vi "observacao_queued.vi"() -> ()   [LabVIEW 2012, in "Shared_160.lvlib"] (continued)
                    n1496 = Get Date/Time In Seconds() -> (seconds since 1Jan1904=w1913:timestamp)
                    n1497 = Add(x=w1913, y=10.0) -> (x+y=w1914:timestamp)
                    n1498 = property on="WeakSel" class="Bool (strict)"("Value"=w1910) -> ()  [unwired: 2 in, 2 out]
                    n1499 = property on="Weak" class="Bool (strict)"("Value"=w1910) -> ()  [unwired: 2 in, 2 out]
                    n1500 = local write "alarm Time"(w1914) -> ()
                    n1501 = property on="Mensage Alarme" class="Str"("Visible"=TRUE) -> ()  [unwired: 2 in, 2 out]
                    n1502 = local write "Flag Alarm"(TRUE ("Flag Alarm")) -> ()
                  }
                }
              }
              event "Medium": Value Change {
                w1917 = u16 6 items=["Alarme", "Atencao", "Erro", "Ocupado", "TBD", "LCB", "Trapeira", "Paravento", "DomoRap", "DomoCW", "DomoCCW", "TBD", "Em movimento", "TBD"] ("NomeStatus")
                n1503 = event-data() -> ("NewVal"=w1918:bool)  [unwired: 1 in, 5 out]
                n1504 = call "Bit Status CUP.vi"("NomeStatus"=w1917) -> ("StatBit"=w1916:bool)
                n1505 = case shown="False" w1916 {
                  tunnel: w1918 -> [w1925 _]
                  frame False {
                    w1920 = u16 4 items=["ZERO", "AH", "DEC", "TUBO", "CUP"] ("Controlador")
                    n1506 = case shown="True" w1925 {
                      tunnel: [0 2] -> w1922
                      tunnel: [w1927 TRUE] -> w1923
                      tunnel: [w1927 FALSE] -> w1921
                      tunnel: ["DESLIGAR" "LIGAR"] -> w1924
                      frame False {
                        w1927 = FALSE
                      }
                      frame True {
                        n1507 = local write "DOME"(FALSE) -> ()
                        n1508 = local write "StatShutter"("Busy to Close" ("Status")) -> ()
                      }
                    }
                    n1509 = property on="Weak" class="Bool (strict)"("Disabled"=w1922) -> ()  [unwired: 2 in, 2 out]
                    n1510 = property on="Strong" class="Bool (strict)"("Disabled"=w1922) -> ()  [unwired: 2 in, 2 out]
                    n1511 = property on="WeakSel" class="Bool (strict)"("Value"=w1921) -> ()  [unwired: 2 in, 2 out]
                    n1512 = property on="MediumSel" class="Bool (strict)"("Value"=w1923) -> ()  [unwired: 2 in, 2 out]
                    n1513 = property on="StrongSel" class="Bool (strict)"("Value"=w1921) -> ()  [unwired: 2 in, 2 out]
                    n1514 = property on="Coude" class="Bool (strict)"("DisabledEnum"=w1922) -> ()  [unwired: 2 in, 2 out]
                    n1515 = property on="CoudeSel" class="Bool (strict)"("Value"=w1921) -> ()  [unwired: 2 in, 2 out]
                    n1516 = call "Monta Comando.vi"("Comando"=w1924, "Dispositivo"="FLAT_LO", "Controlador"=w1920) -> ()  [unwired: 4 in, 3 out]
                  }
                  frame True {
                    w1935 = FALSE ("Medium")
                    n1517 = Get Date/Time In Seconds() -> (seconds since 1Jan1904=w1938:timestamp)
                    n1518 = Add(x=w1938, y=10.0) -> (x+y=w1939:timestamp)
                    n1519 = local write "alarm Time"(w1939) -> ()
                    n1520 = property on="Mensage Alarme" class="Str"("Visible"=TRUE) -> ()  [unwired: 2 in, 2 out]
                    n1521 = local write "Flag Alarm"(TRUE ("Flag Alarm")) -> ()
                    n1522 = property on="Medium" class="Bool (strict)"("Value"=w1935) -> ()  [unwired: 2 in, 2 out]
                    n1523 = property on="MediumSel" class="Bool (strict)"("Value"=w1935) -> ()  [unwired: 2 in, 2 out]
                  }
                }
              }
              event "Strong": Value Change {
                w1942 = u16 6 items=["Alarme", "Atencao", "Erro", "Ocupado", "TBD", "LCB", "Trapeira", "Paravento", "DomoRap", "DomoCW", "DomoCCW", "TBD", "Em movimento", "TBD"] ("NomeStatus")
                n1524 = event-data() -> ("NewVal"=w1943:bool)  [unwired: 1 in, 5 out]
                n1525 = call "Bit Status CUP.vi"("NomeStatus"=w1942) -> ("StatBit"=w1941:bool)
                n1526 = case shown="False" w1941 {
                  tunnel: w1943 -> [w1951 _]
                  frame False {
                    w1944 = u16 4 items=["ZERO", "AH", "DEC", "TUBO", "CUP"] ("Controlador")
                    n1527 = case shown="True" w1951 {
                      tunnel: [FALSE w1959] -> w1946
                      tunnel: [w1952 w1959] -> w1950
                      tunnel: [0 2] -> w1947
                      tunnel: ["DESLIGAR" "LIGAR"] -> w1949
                      tunnel: [w1952 TRUE] -> w1948
                      frame False {
                        w1952 = FALSE
                      }
                      frame True {
                        w1959 = FALSE
                        n1528 = local write "DOME"(FALSE) -> ()
                        n1529 = local write "StatShutter"("Busy to Close" ("Status")) -> ()
                      }
                    }
                    n1530 = property on="Medium" class="Bool (strict)"("Disabled"=w1947) -> ()  [unwired: 2 in, 2 out]
                    n1531 = property on="Weak" class="Bool (strict)"("Disabled"=w1947) -> ()  [unwired: 2 in, 2 out]
                    n1532 = property on="Coude" class="Bool (strict)"("DisabledEnum"=w1947) -> ()  [unwired: 2 in, 2 out]
                    n1533 = property on="WeakSel" class="Bool (strict)"("Value"=w1950) -> ()  [unwired: 2 in, 2 out]
                    n1534 = property on="MediumSel" class="Bool (strict)"("Value"=w1946) -> ()  [unwired: 2 in, 2 out]
                    n1535 = property on="StrongSel" class="Bool (strict)"("Value"=w1948) -> ()  [unwired: 2 in, 2 out]
                    n1536 = property on="CoudeSel" class="Bool (strict)"("Value"=w1946) -> ()  [unwired: 2 in, 2 out]
                    n1537 = call "Monta Comando.vi"("Comando"=w1949, "Dispositivo"="FLAT_HI", "Controlador"=w1944) -> ()  [unwired: 4 in, 3 out]
                  }
                  frame True {
                    w1962 = FALSE ("Strong")
                    n1538 = Get Date/Time In Seconds() -> (seconds since 1Jan1904=w1965:timestamp)
                    n1539 = Add(x=w1965, y=10.0) -> (x+y=w1966:timestamp)
                    n1540 = local write "alarm Time"(w1966) -> ()
                    n1541 = property on="Mensage Alarme" class="Str"("Visible"=TRUE) -> ()  [unwired: 2 in, 2 out]
                    n1542 = local write "Flag Alarm"(TRUE ("Flag Alarm")) -> ()
                    n1543 = property on="StrongSel" class="Bool (strict)"("Value"=w1962) -> ()  [unwired: 2 in, 2 out]
                    n1544 = property on="Strong" class="Bool (strict)"("Value"=w1962) -> ()  [unwired: 2 in, 2 out]
                  }
                }
              }
              event "Coude": Value Change {
                w1969 = u16 6 items=["Alarme", "Atencao", "Erro", "Ocupado", "TBD", "LCB", "Trapeira", "Paravento", "DomoRap", "DomoCW", "DomoCCW", "TBD", "Em movimento", "TBD"] ("NomeStatus")
                n1545 = event-data() -> ("NewVal"=w1970:bool)  [unwired: 1 in, 5 out]
                n1546 = call "Bit Status CUP.vi"("NomeStatus"=w1969) -> ("StatBit"=w1968:bool)
                n1547 = case shown="False" w1968 {
                  tunnel: w1970 -> [w1977 _]
                  frame False {
                    w1971 = u16 4 items=["ZERO", "AH", "DEC", "TUBO", "CUP"] ("Controlador")
                    n1548 = case shown="True" w1977 {
                      tunnel: [FALSE w1986] -> w1974
                      tunnel: [w1979 w1986] -> w1975
                      tunnel: [0 2] -> w1973
                      tunnel: ["DESLIGAR" "LIGAR"] -> w1978
                      tunnel: [w1979 TRUE] -> w1976
                      frame False {
                        w1979 = FALSE
                      }
                      frame True {
                        w1986 = FALSE
                        n1549 = local write "DOME"(FALSE) -> ()
                        n1550 = local write "StatShutter"("Busy to Close" ("Status")) -> ()
                      }
                    }
                    n1551 = property on="StrongSel" class="Bool (strict)"("Value"=w1975) -> ()  [unwired: 2 in, 2 out]
                    n1552 = property on="CoudeSel" class="Bool (strict)"("Value"=w1976) -> ()  [unwired: 2 in, 2 out]
                    n1553 = property on="MediumSel" class="Bool (strict)"("Value"=w1974) -> ()  [unwired: 2 in, 2 out]
                    n1554 = property on="Weak" class="Bool (strict)"("DisabledEnum"=w1973) -> ()  [unwired: 2 in, 2 out]
                    n1555 = property on="Medium" class="Bool (strict)"("DisabledEnum"=w1973) -> ()  [unwired: 2 in, 2 out]
                    n1556 = property on="Strong" class="Bool (strict)"("DisabledEnum"=w1973) -> ()  [unwired: 2 in, 2 out]
                    n1557 = property on="WeakSel" class="Bool (strict)"("Value"=w1974) -> ()  [unwired: 2 in, 2 out]
                    n1558 = call "Monta Comando.vi"("Comando"=w1978, "Dispositivo"="FLAT_COUDE", "Controlador"=w1971) -> ()  [unwired: 4 in, 3 out]
                  }
                  frame True {
                    w1989 = FALSE ("Coude")
                    n1559 = Get Date/Time In Seconds() -> (seconds since 1Jan1904=w1992:timestamp)
                    n1560 = Add(x=w1992, y=10.0) -> (x+y=w1993:timestamp)
                    n1561 = local write "alarm Time"(w1993) -> ()
                    n1562 = property on="Mensage Alarme" class="Str"("Visible"=TRUE) -> ()  [unwired: 2 in, 2 out]
                    n1563 = local write "Flag Alarm"(TRUE ("Flag Alarm")) -> ()
                    n1564 = property on="CoudeSel" class="Bool (strict)"("Value"=w1989) -> ()  [unwired: 2 in, 2 out]
                    n1565 = property on="Coude" class="Bool (strict)"("Value"=w1989) -> ()  [unwired: 2 in, 2 out]
                  }
                }
              }
            }
            n1566 = disable-structure shown="Disabled" {
              frame Disabled {
                w1889 = u16 4 items=["ZERO", "AH", "DEC", "TUBO", "CUP"] ("Controlador")
                n1567 = call "Monta Comando.vi"("Comando"="FECHAR", "Dispositivo"="TRAPEIRA" ("Comando"), "Controlador"=w1889) -> ()  [unwired: 4 in, 3 out]
              }
              frame Enabled {
              }
            }
          }
          frame "LIST" {
            n1568 = stacked-sequence {
              frame #0 {
                # "Muda nome do controle de RA para AH se MAFmax == 100"
                n1569 = case shown="True" "SET coord" {
                  frame False {
                  }
                  frame True {
                    n1570 = stacked-sequence {
                      frame #0 {
                        w2010 = "2000"
                        # "Valores aux para Detectar Edição"
                        n1571 = local read "Multicolumn Listbox"() -> (w2017:i32[])
                        n1572 = property on="Multicolumn Listbox" class="MCListbox (strict)"() -> ("Item Names"=w2015:string[][])  [unwired: 2 in, 2 out]
                        n1573 = Index Array(array=w2017, index=0) -> (element=w2014:i32)
                        n1574 = local write "FLAG SET COORD"(TRUE ("FLAG_MAG")) -> ()
                        n1575 = Index Array(array=w2015, index (row)=w2014) -> (element=w2013:string[])  [unwired: 1 in]
                        n1576 = Index Array(array=w2013, index #1=0 ("index")) -> (element #1=w2006:string, element #2=w2004:string, element #3=w2005:string, element #4=w2007:string, element #5=w2009:string, element #6=w2008:string)  [unwired: 5 in]
                        "RA AUX" <- w2004
                        "AUX EDITA Name" <- w2006
                        "AUX EDITA RA" <- w2004
                        "AUX EDITA DEC" <- w2005
                        "AUX EDITA PMRA" <- w2009
                        "AUX EDITA PMDEC" <- w2008
                        n1577 = local write "StrPointObjPMRA"(w2009) -> ()
                        n1578 = local write "StrPointObjPMDEC"(w2008) -> ()
                        n1579 = local write "StrPointObjName"(w2006) -> ()
                        n1580 = local write "StrPointObjRA"(w2004) -> ()
                        n1581 = local write "StrPointObjDEC"(w2005) -> ()
                        n1582 = local write "MAG"(w2007) -> ()
                        n1583 = local write "StrPointObjEpoch"(w2010) -> ()
                        "EPOCH AUX" <- w2010
                        "AUX EDITA EPOCH" <- w2010
                      }
                      frame #1 {
                        n1584 = case shown="True" "Case Constant\n(See Context Help) 7" {
                          frame False {
                          }
                          frame True {
                            # "Ao clicar SET COORD, fechar a aba LIST e abrir a aba POINTING"
                            n1585 = local write "Setup, Pointing & Guiding"(T2."POINTING" ("Setup, Pointing & Guiding")) -> ()
                          }
                        }
                      }
                    }
                  }
                }
                n1586 = case shown="True" "Clear ALL" {
                  frame False {
                  }
                  frame True {
                    n1587 = Two Button Dialog(message="Will you clear All Table?") -> (T button?=w2020:bool)  [unwired: 2 in]
                    n1588 = case shown="True" w2020 {
                      frame False {
                      }
                      frame True {
                        w2022 = string[][] [] ("Item Names")
                        # "Limpa a Tabela Inteira"
                        n1589 = property on="Multicolumn Listbox" class="MCListbox (strict)"("Item Names"=w2022) -> ()  [unwired: 2 in, 2 out]
                        n1590 = local write "subarray"(w2022) -> ()
                      }
                    }
                  }
                }
                n1591 = local read "MAG Max"() -> (w1996:dbl)
                n1592 = Equal?(x=100.0, y=w1996) -> (x = y?=w1995:bool)
                n1593 = case shown="False" w1995 {
                  frame False {
                    n1594 = flat-sequence {
                      frame #0 {
                        w2000 = FALSE
                        n1595 = property on="RA Max" class="DigNum (strict)"("Caption.Visible"=w2000) -> ()  [unwired: 2 in, 2 out]
                        n1596 = property on="RA Min" class="DigNum (strict)"("Caption.Visible"=w2000) -> ()  [unwired: 2 in, 2 out]
                      }
                      frame #1 {
                        w2001 = TRUE
                        n1597 = property on="RA Min" class="DigNum (strict)"("Label.Visible"=w2001) -> ()  [unwired: 2 in, 2 out]
                        n1598 = property on="RA Max" class="DigNum (strict)"("Label.Visible"=w2001) -> ()  [unwired: 2 in, 2 out]
                      }
                    }
                  }
                  frame True {
                    n1599 = flat-sequence {
                      frame #0 {
                        w2002 = FALSE
                        n1600 = property on="RA Max" class="DigNum (strict)"("Label.Visible"=w2002) -> ()  [unwired: 2 in, 2 out]
                        n1601 = property on="RA Min" class="DigNum (strict)"("Label.Visible"=w2002) -> ()  [unwired: 2 in, 2 out]
                      }
                      frame #1 {
                        w2003 = TRUE
                        n1602 = property on="RA Min" class="DigNum (strict)"("Caption.Visible"=w2003) -> ()  [unwired: 2 in, 2 out]
                        n1603 = property on="RA Max" class="DigNum (strict)"("Caption.Visible"=w2003) -> ()  [unwired: 2 in, 2 out]
                      }
                    }
                  }
                }
              }
              frame #1 {
                # "MUDANÇA:\nUPLOAD carrega\ncatálogo usuário"
                n1604 = case shown="True" "Upload" {
                  frame False {
                  }
                  frame True {
                    n1605 = File Dialog() -> (0:w2028:errorcluster, 1:w2030:bool, 3:w2029:path)  [unwired: 7 in, 1 out]
                    n1606 = Unbundle(w2028) -> ("status"=w2027:bool)  [unwired: 2 out]
                    n1607 = Not(x=w2027) -> (.not. x?=w2025:bool)
                    n1608 = And(x=w2030, y=w2025) -> (x .and. y?=w2026:bool)
                    n1609 = case shown="False" w2026 {
                      tunnel: w2029 -> [w2033 _]
                      frame False {
                        w2034 = 0 ("Slide")
                        # "Abre Arquivo Escolhido"
                        n1610 = Strip Path(path=w2033) -> (name=w2031:string)  [unwired: 1 out]
                        n1611 = Path To String(path=w2033) -> (string=w2038:string)
                        n1612 = local write "List File"(w2031) -> ()
                        n1613 = call "leexel.vi"("path"=w2038) -> ("array 5"=w2032:string[][])  [unwired: 4 in]
                        n1614 = local write "Slide"(w2034) -> ()
                        n1615 = local write "subarray"(w2032) -> ()
                        n1616 = Array Subset(array=w2032, index (row)=w2034, length (row)=10 ("length"), index (col)=w2034, length (col)=8 ("index")) -> (w2035:string[][])
                        n1617 = property on="Multicolumn Listbox" class="MCListbox (strict)"("Item Names"=w2035) -> ()  [unwired: 2 in, 2 out]
                      }
                      frame True {
                      }
                    }
                  }
                }
                n1618 = case shown="True" "Save AS" {
                  frame False {
                  }
                  frame True {
                    n1619 = File Dialog() -> (0:w2039:errorcluster, 1:w2041:bool, 3:w2040:path)  [unwired: 7 in, 1 out]
                    n1620 = Unbundle(w2039) -> ()  [unwired: 3 out]
                    n1621 = case shown="False" w2041 {
                      tunnel: w2040 -> [w2043 _]
                      frame False {
                        # "Salva Arquivo Escolhido"
                        n1622 = Path To String(path=w2043) -> (string=w2044:string)
                        n1623 = case shown="True" "Case Constant\n(See Context Help) 8" {
                          tunnel: w2044 -> [_ w2046]
                          frame False {
                          }
                          frame True {
                            n1624 = local read "subarray"() -> (w2045:string[][])
                            n1625 = call "salvaexel.vi"("appended array"=w2045, "file name p/ exell"=w2046) -> ()  [unwired: 1 in, 1 out]
                          }
                        }
                      }
                      frame True {
                      }
                    }
                  }
                }
              }
              frame #2 {
                # "Acerta Posição do Slide"
                n1626 = local read "Tot Linhas"() -> (w2051:i32)
                n1627 = Multiply(x="Slide", y=w2051) -> (x*y=w2050:dbl)
                n1628 = Divide(x=w2050, y=24.0) -> (x/y=w2048:dbl)
                n1629 = case shown="True" "Save" {
                  frame False {
                  }
                  frame True {
                    w2102 = "C:\\TCS\\ARQUIVOS\\List.lst"
                    # "Cria e Lê arquivo\nonde voce está\ntrabalhando"
                    n1630 = String To Path(string=w2102) -> (path=w2101:path)
                    n1631 = stacked-sequence {
                      tunnel: w2101 -> [w2103 _]
                      tunnel: w2102 -> [_ w2105]
                      frame #0 {
                        # "Apaga o arquivo"
                        n1632 = Delete(path (use dialog)=w2103) -> ()  [unwired: 4 in, 3 out]
                      }
                      frame #1 {
                        # "Salva a lista"
                        n1633 = local read "subarray"() -> (w2104:string[][])
                        n1634 = call "salvaexel.vi"("appended array"=w2104, "file name p/ exell"=w2105) -> ()  [unwired: 1 in, 1 out]
                      }
                    }
                  }
                }
                n1635 = Not Equal?(x=w2048, y="Slide old") -> (x != y?=w2054:bool)
                n1636 = case shown="True" "Open BSC" {
                  frame False {
                  }
                  frame True {
                    n1637 = stacked-sequence {
                      frame #0 {
                        w2107 = FALSE
                        # "MUDANÇA:\nUPLOAD carrega\ncatálogo usuário"
                        # "Faz Aparecer os Botões"
                        n1638 = property on="Delete" class="Bool"("Visible"=w2107) -> ()  [unwired: 2 in, 2 out]
                        n1639 = property on="EDIT" class="Bool"("Visible"=w2107) -> ()  [unwired: 2 in, 2 out]
                        n1640 = property on="Clear ALL" class="Bool"("Visible"=w2107) -> ()  [unwired: 2 in, 2 out]
                        n1641 = property on="Save AS" class="Bool"("Visible"=w2107) -> ()  [unwired: 2 in, 2 out]
                        n1642 = property on="Save" class="Bool"("Visible"=w2107) -> ()  [unwired: 2 in, 2 out]
                        n1643 = property on="Insert" class="Bool"("Visible"=w2107) -> ()  [unwired: 2 in, 2 out]
                        n1644 = property on="Upload" class="Bool"("Visible"=TRUE) -> ()  [unwired: 2 in, 2 out]
                      }
                      frame #1 {
                        w2115 = 0 ("Slide")
                        w2109 = "C:\\TCS\\ARQUIVOS\\BSC_08.txt"
                        # "Cria e Lê arquivo\nonde voce está\ntrabalhando"
                        n1645 = local write "Slide"(w2115) -> ()
                        n1646 = call "leexel.vi"("path"=w2109) -> ("array 5"=w2113:string[][])  [unwired: 4 in]
                        "subarray" <- w2113
                        n1647 = Array Subset(array=w2113, index (row)=w2115, length (row)=11 ("length"), index (col)=w2115, length (col)=8 ("index")) -> (w2116:string[][])
                        n1648 = Array Size(array=w2113) -> (size(s)=w2114:i32[])
                        n1649 = String To Path(string=w2109) -> (path=w2110:path)
                        n1650 = property on="Multicolumn Listbox" class="MCListbox (strict)"("Item Names"=w2116) -> ()  [unwired: 2 in, 2 out]
                        n1651 = Strip Path(path=w2110) -> (name=→"List File":string)  [unwired: 1 out]
                        n1652 = Index Array(array=w2114, index=0) -> (element=→"Tot Linhas":i32)
                        "Saida Path string" <- w2109
                      }
                      frame #2 {
                        n1653 = local read "Tot Linhas"() -> (w2127:i32)
                        n1654 = Quotient & Remainder(x=10000, y=w2127) -> (floor(x/y)=w2125:i32)  [unwired: 1 out]
                        n1655 = Divide(x=w2125, y=1000) -> (x/y=w2122:dbl)
                        n1656 = Multiply(x=w2122, y=24.0) -> (x*y=w2123:dbl)
                        n1657 = property on="Slide" class="Slide (strict)"("Data Entry Limits:Increment"=w2123) -> ()  [unwired: 2 in, 2 out]
                        "ScaleMax" <- "24" ("ScaleMax")
                        "ScaleMin" <- "0" ("ScaleMin")
                      }
                    }
                  }
                }
                n1658 = case shown="True" w2054 {
                  tunnel: w2048 -> [_ w2059]
                  frame False {
                  }
                  frame True {
                    n1659 = stacked-sequence {
                      seq-local: [w2063 _] -> [_ w2068]
                      tunnel: w2059 -> [w2064 _]
                      frame #0 {
                        # "Previne estouro\nda planilha"
                        n1660 = local read "Tot Linhas"() -> (w2062:i32)
                        n1661 = Subtract(x=w2062, y=10) -> (x-y=w2060:i32)
                        n1662 = Greater Or Equal?(x=w2064, y=w2060) -> (x >= y?=w2065:bool)
                        n1663 = case shown="False" w2065 {
                          tunnel: [w2066 w2067] -> w2063
                          tunnel: w2060 -> [_ w2067]
                          tunnel: w2064 -> [w2066 _]
                          frame False {
                          }
                          frame True {
                          }
                        }
                      }
                      frame #1 {
                        n1664 = local read "subarray"() -> (w2070:string[][])
                        n1665 = local write "Slide old"(w2068) -> ()
                        n1666 = Array Subset(array=w2070, index (row)=w2068, length (row)=11 ("length"), index (col)=0 ("index"), length (col)=8 ("index")) -> (w2069:string[][])
                        n1667 = property on="Multicolumn Listbox" class="MCListbox (strict)"("Item Names"=w2069) -> ()  [unwired: 2 in, 2 out]
                      }
                    }
                  }
                }
                n1668 = property on="Multicolumn Listbox" class="MCListbox (strict)"("Selection Color"=u32 10336195) -> ()  [unwired: 2 in, 2 out]
                n1669 = case shown="True" "Delete" {
                  frame False {
                  }
                  frame True {
                    n1670 = local read "Multicolumn Listbox"() -> (w2080:i32[])
                    n1671 = Index Array(array=w2080, index=0) -> (element=w2074:i32)
                    n1672 = Number To Decimal String(number=w2074) -> (decimal integer string=w2077:string)  [unwired: 1 in]
                    n1673 = Concatenate Strings("Delete Line Number: " ("string"), w2077) -> (w2075:string)
                    n1674 = Two Button Dialog(message=w2075) -> (T button?=w2076:bool)  [unwired: 2 in]
                    n1675 = case shown="True" w2076 {
                      tunnel: w2074 -> [_ w2081]
                      frame False {
                      }
                      frame True {
                        n1676 = stacked-sequence {
                          tunnel: w2081 -> [w2085 _]
                          frame #0 {
                            # "Apaga a Coluna Escolhida"
                            n1677 = property on="Multicolumn Listbox" class="MCListbox (strict)"() -> ("Item Names"=w2088:string[][])  [unwired: 2 in, 2 out]
                            n1678 = local read "Slide"() -> (w2086:dbl)
                            n1679 = local read "subarray"() -> (w2083:string[][])
                            n1680 = Add(x=w2085, y=w2086) -> (x+y=w2084:dbl)
                            n1681 = Delete From Array(array=w2088, index (row)=w2085) -> (array with subset deleted=w2087:string[][])  [unwired: 2 in, 1 out]
                            n1682 = Delete From Array(array=w2083, index (row)=w2084) -> (array with subset deleted=w2082:string[][])  [unwired: 2 in, 1 out]
                            n1683 = local write "subarray"(w2082) -> ()
                            n1684 = property on="Multicolumn Listbox" class="MCListbox (strict)"("Item Names"=w2087) -> ()  [unwired: 2 in, 2 out]
                          }
                          frame #1 {
                            # "Volta para a coluna Zero"
                            n1685 = local write "Multicolumn Listbox"(i32[] [0] ("Multicolumn Listbox")) -> ()
                          }
                        }
                      }
                    }
                  }
                }
                n1686 = case shown="True" "Insert" {
                  frame False {
                  }
                  frame True {
                    n1687 = stacked-sequence {
                      seq-local: [w2091 _ _] -> [_ w2093 _]
                      seq-local: [w2090 _ _] -> [_ w2092 _]
                      frame #0 {
                        n1688 = call "Tela_Set_Coordenadas.vi"() -> ("Saída"=w2091:bool, "Val Saída"=w2090:string[])  [unwired: 4 in]
                      }
                      frame #1 {
                        n1689 = case shown="True" w2093 {
                          tunnel: w2092 -> [_ w2094]
                          frame False {
                          }
                          frame True {
                            # "Insere Linha Preenchida"
                            n1690 = local read "subarray"() -> (w2096:string[][])
                            n1691 = property on="Multicolumn Listbox" class="MCListbox (strict)"() -> ("Item Names"=w2098:string[][])  [unwired: 2 in, 2 out]
                            n1692 = Build Array (concatenate)(w2098, w2094) -> (w2097:string[][])
                            n1693 = Build Array (concatenate)(w2096, w2094) -> (w2095:string[][])
                            n1694 = property on="Multicolumn Listbox" class="MCListbox (strict)"("Item Names"=w2097) -> ()  [unwired: 2 in, 2 out]
                            n1695 = local write "subarray"(w2095) -> ()
                          }
                        }
                      }
                      frame #2 {
                        # "Depois de inserir um novo objeto na tabela,\n com o comando INSERT, mudar o objeto \nselecionado para esse novo registro."
                        n1696 = property on="Multicolumn Listbox" class="MCListbox (strict)"() -> ("Number of Rows"=w2100:u32)  [unwired: 2 in, 2 out]
                        n1697 = Build Array(w2100) -> (w2099:u32[])
                        n1698 = local write "Multicolumn Listbox"(w2099) -> ()
                      }
                    }
                  }
                }
              }
              frame #3 {
                # "Editar a Lista"
                n1699 = case shown="True" "Open" {
                  frame False {
                  }
                  frame True {
                    n1700 = stacked-sequence {
                      frame #0 {
                        w2130 = TRUE
                        # "Faz Aparecer os Botões"
                        n1701 = property on="Delete" class="Bool"("Visible"=w2130) -> ()  [unwired: 2 in, 2 out]
                        n1702 = property on="EDIT" class="Bool"("Visible"=w2130) -> ()  [unwired: 2 in, 2 out]
                        n1703 = property on="Clear ALL" class="Bool"("Visible"=w2130) -> ()  [unwired: 2 in, 2 out]
                        n1704 = property on="Upload" class="Bool"("Visible"=w2130) -> ()  [unwired: 2 in, 2 out]
                        n1705 = property on="Save AS" class="Bool"("Visible"=w2130) -> ()  [unwired: 2 in, 2 out]
                        n1706 = property on="Save" class="Bool"("Visible"=w2130) -> ()  [unwired: 2 in, 2 out]
                        n1707 = property on="Insert" class="Bool"("Visible"=w2130) -> ()  [unwired: 2 in, 2 out]
                      }
                      frame #1 {
                        w2138 = 0 ("Slide")
                        w2134 = "C:\\TCS\\ARQUIVOS\\List.lst"
                        n1708 = local write "Saida Path string"(w2134) -> ()
                        n1709 = local write "Slide"(w2138) -> ()
                        n1710 = String To Path(string=w2134) -> (path=w2141:path)
                        n1711 = call "leexel.vi"("path"=w2134) -> ("array 5"=w2133:string[][])  [unwired: 4 in]
                        n1712 = Strip Path(path=w2141) -> (name=w2140:string)  [unwired: 1 out]
                        n1713 = local write "subarray"(w2133) -> ()
                        n1714 = local write "List File"(w2140) -> ()
                        n1715 = Array Subset(array=w2133, index (row)=w2138, length (row)=10 ("length"), index (col)=w2138, length (col)=8 ("index")) -> (w2137:string[][])
                        n1716 = Array Size(array=w2133) -> (size(s)=w2131:i32[])
                        n1717 = property on="Multicolumn Listbox" class="MCListbox (strict)"("Item Names"=w2137) -> ()  [unwired: 2 in, 2 out]
                        n1718 = Index Array(array=w2131, index=0) -> (element=w2132:i32)
                        n1719 = local write "Tot Linhas"(w2132) -> ()
                      }
                      frame #2 {
                        w2142 = ""
                        n1720 = local read "Tot Linhas"() -> (w2149:i32)
                        n1721 = Quotient & Remainder(x=10000, y=w2149) -> (floor(x/y)=w2147:i32)  [unwired: 1 out]
                        n1722 = Divide(x=w2147, y=1000) -> (x/y=w2144:dbl)
                        n1723 = Multiply(x=w2144, y=24.0) -> (x*y=w2145:dbl)
                        n1724 = local write "ScaleMin"(w2142) -> ()
                        n1725 = local write "ScaleMax"(w2142) -> ()
                        n1726 = property on="Slide" class="Slide (strict)"("Data Entry Limits:Increment"=w2145) -> ()  [unwired: 2 in, 2 out]
                      }
                    }
                  }
                }
                n1727 = case shown="True" "EDIT" {
                  frame False {
                  }
                  frame True {
                    (unwired) "Edit the marked Line and soon after presses SAVE"
                    n1728 = call "Edita_lista.vi"() -> ("lista Auxiliar"=w2150:string[][])  [unwired: 5 in]
                    n1729 = property on="Multicolumn Listbox" class="MCListbox (strict)"("Item Names"=w2150) -> ()  [unwired: 2 in, 2 out]
                  }
                }
              }
              frame #4 {
                n1730 = case shown="True" "Filter RA" {
                  frame False {
                  }
                  frame True {
                    n1731 = while {
                      shift-right: [w2153] -> _
                      shift-left: "inicio" -> [w2155]
                      stop <- w2154 stop-if-true
                      n1732 = case shown="\"filtra\"" w2155 {
                        tunnel: [FALSE w2205 TRUE TRUE] -> w2154
                        tunnel: [w2175 w2206 "fim" "fim"] -> w2153
                        frame "inicio" {
                          # "RAmin"
                          # "RAmax"
                          # "Testa se:\n| Ramax - Ramin | >=1\n|Decmax -Decmin | >=1\n|Magmax -Magmin | >=1"
                          n1733 = local read "MAG Max"() -> (w2169:dbl)
                          n1734 = local read "MAG Min"() -> (w2184:dbl)
                          n1735 = Equal?(x=100.0, y=w2169) -> (x = y?=w2161:bool)
                          n1736 = Subtract(x=w2169, y=w2184) -> (x-y=w2181:dbl)
                          n1737 = case shown="True" w2161 {
                            tunnel: "RA Min" -> [w2189 w2197]
                            tunnel: [w2189 w2196] -> w2156
                            tunnel: "RA Max" -> [w2188 w2198]
                            tunnel: [w2188 w2193] -> w2157
                            frame False {
                            }
                            frame True {
                              w2202 = 24 ("RA Max")
                              # "12h/PI()"
                              # "TS, rad"
                              # "TS, hora"
                              # "RAmin"
                              # "RAmax"
                              # "AHmax"
                              # "AHmin"
                              # "MUDANÇA 7/4/2011:\nSe MAGmax >= 100,\ntratar RA como AH."
                              n1738 = global read "Global_Telescopio.vi" "Sideral Time"() -> (w2192:dbl)
                              n1739 = Multiply(x=w2192, y=3.8197) -> (x*y=w2191:dbl)
                              n1740 = To Long Integer(number=w2191) -> (32bit integer=w2199:i32)
                              n1741 = Subtract(x=w2199, y=w2198) -> (x-y=w2195:i32)
                              n1742 = Subtract(x=w2199, y=w2197) -> (x-y=w2194:i32)
                              n1743 = Add(x=w2202, y=w2195) -> (x+y=w2201:i32)
                              n1744 = Less Than 0?(x=w2195) -> (x < 0?=w2204:bool)
                              n1745 = Add(x=w2202, y=w2194) -> (x+y=w2200:i32)
                              n1746 = Less Than 0?(x=w2194) -> (x < 0?=w2203:bool)
                              n1747 = Select(t=w2201, s=w2204, f=w2195) -> (s? t:f=w2196:i32)
                              n1748 = Select(t=w2200, s=w2203, f=w2194) -> (s? t:f=w2193:i32)
                            }
                          }
                          n1749 = Less?(x=w2181, y=1.0) -> (x < y?=w2178:bool)
                          n1750 = local read "DEC Max"() -> (w2186:i32)
                          n1751 = local read "DEC Min"() -> (w2185:i32)
                          n1752 = local write "RA Min 2"(w2156) -> ()
                          n1753 = local write "RA Max 2"(w2157) -> ()
                          n1754 = Less?(x=w2157, y=w2156) -> (x < y?=w2162:bool)
                          "FiltroDuplo" <- w2162
                          n1755 = Equal?(x=w2157, y=w2156) -> (x = y?=w2160:bool)
                          n1756 = Add(x=w2157, y=24 ("RA Max")) -> (x+y=w2166:i32)
                          n1757 = Subtract(x=w2166, y=w2156) -> (x-y=w2165:i32)
                          n1758 = Subtract(x=w2186, y=w2185) -> (x-y=w2183:i32)
                          n1759 = Greater?(x=w2165, y=12) -> (0:w2163:bool)
                          n1760 = Less?(x=w2183, y=1) -> (x < y?=w2179:bool)
                          n1761 = And(x=w2163, y=w2162) -> (x .and. y?=w2170:bool)
                          n1762 = control-ref of="Erro"() -> (w2172:refnum<vi>)
                          n1763 = Compound Arithmetic op=OR(w2170, w2160, w2179, w2178) -> (w2177:bool)
                          n1764 = property class="Bool (strict)"(reference=w2172, "Boolean Text.Text"="WAIT") -> ()  [unwired: 1 in, 2 out]
                          n1765 = Select(t="erro", s=w2177, f="filtra") -> (s? t:f=w2175:string)
                          "Erro" <- FALSE ("Fim")
                        }
                        frame "filtra" {
                          n1766 = stacked-sequence {
                            seq-local: [w2210 _ _ _] -> [_ w2253 _ _]
                            seq-local: [_ w2254 _ _] -> [_ _ w2273 _]
                            seq-local: [_ _ w2274 _] -> [_ _ _ w2299]
                            tunnel: [_ _ _ "fim"] -> w2206
                            tunnel: [_ _ _ FALSE] -> w2205
                            frame #0 {
                              n1767 = property on="EDIT" class="Bool"() -> ("Visible"=w2207:bool)  [unwired: 2 in, 2 out]
                              n1768 = case shown="True" w2207 {
                                tunnel: ["C:\\TCS\\ARQUIVOS\\BSC_08.txt" "C:\\TCS\\ARQUIVOS\\List.lst"] -> w2209
                                frame False {
                                }
                                frame True {
                                }
                              }
                              n1769 = call "leexel.vi"("path"=w2209) -> ("array 5"=w2208:string[][])  [unwired: 4 in]
                              n1770 = Index Array(array=w2208, index (col)=1 ("disabled index (col)")) -> (element=w2212:string[])  [unwired: 1 in]
                              n1771 = for {
                                tunnel: w2212 -> [w2228] mode=indexing
                                shift-right: [w2222] -> w2210
                                shift-left: string[][] [] ("Item Names") -> [w2224]
                                tunnel: w2208 -> [w2221] mode=indexing
                                # "Filtro de RA"
                                n1772 = local read "FiltroDuplo"() -> (w2220:bool)
                                n1773 = String Subset(string=w2228, offset (0)=0, length (rest)=2 ("length (rest)")) -> (substring=w2225:string)
                                n1774 = Decimal String To Number(string=w2225) -> (number=w2219:i32)  [unwired: 2 in, 1 out]
                                n1775 = case shown="False" w2220 {
                                tunnel: "RA Max 2" -> [w2233 w2238]
                                tunnel: "RA Min 2" -> [w2232 w2235]
                                tunnel: [w2231 w2240] -> w2223
                                tunnel: w2219 -> [w2230 w2239]
                                tunnel: [FALSE w2234] -> w2218
                                frame False {
                                n1776 = In Range and Coerce(upper limit=w2233, x=w2230, lower limit=w2232) -> (In Range?=w2231:bool)  [unwired: 1 out]
                                }
                                frame True {
                                n1777 = In Range and Coerce(upper limit=w2238, x=w2239, lower limit=0 ("upper limit")) -> (In Range?=w2241:bool)  [unwired: 1 out]
                                n1778 = In Range and Coerce(upper limit=24 ("lower limit"), x=w2239, lower limit=w2235) -> (In Range?=w2234:bool)  [unwired: 1 out]
                                n1779 = Or(x=w2241, y=w2234) -> (x .or. y?=w2240:bool)
                                }
                                }
                                n1780 = case shown="True" w2223 {
                                tunnel: w2224 -> [w2242 w2246]
                                tunnel: [w2242 w2245] -> w2222
                                tunnel: w2221 -> [_ w2244]
                                tunnel: w2218 -> [_ w2243]
                                frame False {
                                }
                                frame True {
                                n1781 = case shown="False" w2243 {
                                tunnel: w2246 -> [w2249 w2251]
                                tunnel: [w2248 w2250] -> w2245
                                tunnel: w2244 -> [w2247 w2252]
                                frame False {
                                n1782 = Build Array (concatenate)(w2249, w2247) -> (w2248:string[][])
                                }
                                frame True {
                                n1783 = Build Array (concatenate)(w2252, w2251) -> (w2250:string[][])
                                }
                                }
                                }
                                }
                              }
                            }
                            frame #1 {
                              # "Filtro de DEC"
                              n1784 = Index Array(array=w2253, index (col)=2 ("disabled index (col)")) -> (element=w2256:string[])  [unwired: 1 in]
                              n1785 = for {
                                tunnel: w2256 -> [w2268] mode=indexing
                                shift-right: [w2261] -> w2254
                                shift-left: string[][] [] ("Item Names") -> [w2263]
                                tunnel: w2253 -> [w2260] mode=indexing
                                n1786 = String Subset(string=w2268, offset (0)=0, length (rest)=3 ("length (rest)")) -> (substring=w2265:string)
                                n1787 = Decimal String To Number(string=w2265) -> (number=w2264:i32)  [unwired: 2 in, 1 out]
                                n1788 = In Range and Coerce(upper limit="DEC Max", x=w2264, lower limit="DEC Min") -> (In Range?=w2262:bool)  [unwired: 1 out]
                                n1789 = case shown="True" w2262 {
                                tunnel: w2263 -> [w2269 w2272]
                                tunnel: [w2269 w2271] -> w2261
                                tunnel: w2260 -> [_ w2270]
                                frame False {
                                }
                                frame True {
                                n1790 = Build Array (concatenate)(w2272, w2270) -> (w2271:string[][])
                                }
                                }
                              }
                            }
                            frame #2 {
                              # "Filtro de MAG"
                              n1791 = Index Array(array=w2273, index (col)=3 ("disabled index (col)")) -> (element=w2276:string[])  [unwired: 1 in]
                              n1792 = for {
                                tunnel: w2276 -> [w2278] mode=indexing
                                shift-right: [w2282] -> w2274
                                shift-left: string[][] [] ("Item Names") -> [w2286]
                                tunnel: w2273 -> [w2284] mode=indexing
                                n1793 = Fract/Exp String To Number(use system decimal point (T)=FALSE, string=w2278) -> (number=w2281:dbl)  [unwired: 2 in, 1 out]
                                n1794 = In Range and Coerce(upper limit="MAG Max", x=w2281, lower limit="MAG Min") -> (In Range?=w2285:bool)  [unwired: 1 out]
                                n1795 = case shown="True" w2285 {
                                tunnel: w2286 -> [w2287 w2290]
                                tunnel: [w2287 w2289] -> w2282
                                tunnel: w2284 -> [_ w2288]
                                frame False {
                                }
                                frame True {
                                n1796 = Build Array (concatenate)(w2290, w2288) -> (w2289:string[][])
                                }
                                }
                              }
                            }
                            frame #3 {
                              w2291 = 0 ("index")
                              n1797 = local write "subarray"(w2299) -> ()
                              n1798 = Array Size(array=w2299) -> (size(s)=w2311:i32[])
                              n1799 = Index Array(array=w2311, index=0) -> (element=w2304:i32)
                              n1800 = local write "Tot Linhas"(w2304) -> ()
                              n1801 = local write "Slide old"(w2291) -> ()
                              n1802 = local write "Slide"(w2291) -> ()
                              n1803 = Array Subset(array=w2299, index (row)=w2291, length (row)=11 ("length"), index (col)=0 ("index"), length (col)=8 ("index")) -> (w2300:string[][])
                              n1804 = property on="Multicolumn Listbox" class="MCListbox (strict)"("Item Names"=w2300) -> ()  [unwired: 2 in, 2 out]
                              n1805 = Quotient & Remainder(x=10000, y=w2304) -> (floor(x/y)=w2308:i32)  [unwired: 1 out]
                              n1806 = Divide(x=w2308, y=1000) -> (x/y=w2306:dbl)
                              n1807 = Multiply(x=w2306, y=24.0) -> (x*y=w2293:dbl)
                              n1808 = Decrement(x=w2293) -> (x-1=w2292:dbl)
                              n1809 = control-ref of="Erro"() -> (w2295:refnum<vi>)
                              n1810 = property class="Bool (strict)"(reference=w2295, "Boolean Text.Text"="") -> ()  [unwired: 1 in, 2 out]
                              n1811 = property on="Slide" class="Slide (strict)"("Data Entry Limits:Increment"=w2292) -> ()  [unwired: 2 in, 2 out]
                              n1812 = local write "Erro"(FALSE ("Erro")) -> ()
                            }
                          }
                        }
                        frame "erro", Default {
                          n1813 = control-ref of="Erro"() -> (w2313:refnum<vi>)
                          n1814 = property class="Bool (strict)"(reference=w2313, "Boolean Text.Text"="ERROR") -> ()  [unwired: 1 in, 2 out]
                          n1815 = local write "Erro"(TRUE ("Erro")) -> ()
                        }
                        frame "fim" {
                          n1816 = local read "RA Max 2"() -> (w2318:i32)
                          n1817 = local read "RA Min 2"() -> (w2317:i32)
                          n1818 = Number To Decimal String(number=w2317) -> (decimal integer string=w2320:string)  [unwired: 1 in]
                          n1819 = Number To Decimal String(number=w2318) -> (decimal integer string=w2319:string)  [unwired: 1 in]
                          n1820 = local write "ScaleMin"(w2320) -> ()
                          n1821 = local write "ScaleMax"(w2319) -> ()
                        }
                      }
                    }
                  }
                }
              }
            }
          }
          frame " INSTRUMENT " {
            n1822 = case shown="\"Casseg.\"" "TabInstrumento" {
              frame "Casseg." {
                w2334 = u16 13 items=["Alarme", "Atencao", "Erro", "Ocupado", "PosSecund", "PosConj#3", "MovFoco", "MovCjto#3", "Mov#4", "Mov#3", "Mov#2", "EspLamp", "HE", "NE", "EspLampRepouso", "EspLampCalibra"] ("NomeStatus")
                w2333 = u16 12 items=["Alarme", "Atencao", "Erro", "Ocupado", "PosSecund", "PosConj#3", "MovFoco", "MovCjto#3", "Mov#4", "Mov#3", "Mov#2", "EspLamp", "HE", "NE", "EspLampRepouso", "EspLampCalibra"] ("NomeStatus")
                w2335 = u16 15 items=["Alarme", "Atencao", "Erro", "Ocupado", "PosSecund", "PosConj#3", "MovFoco", "MovCjto#3", "Mov#4", "Mov#3", "Mov#2", "EspLamp", "HE", "NE", "EspLampRepouso", "EspLampCalibra"] ("NomeStatus")
                w2336 = u16 14 items=["Alarme", "Atencao", "Erro", "Ocupado", "PosSecund", "PosConj#3", "MovFoco", "MovCjto#3", "Mov#4", "Mov#3", "Mov#2", "EspLamp", "HE", "NE", "EspLampRepouso", "EspLampCalibra"] ("NomeStatus")
                w2337 = u16 11 items=["Alarme", "Atencao", "Erro", "Ocupado", "PosSecund", "PosConj#3", "MovFoco", "MovCjto#3", "Mov#4", "Mov#3", "Mov#2", "EspLamp", "HE", "NE", "EspLampRepouso", "EspLampCalibra"] ("NomeStatus")
                # "Cassegrain"
                n1823 = event shown="[3] \"Sent_EspLampCass\": Value Change" {
                  selector: _ -> [_ _ _ _]
                  dyn-events: _ -> [_ _ _ _]
                  timeout: 10 -> [_ _ _ _]
                  event Timeout {
                    n1824 = event-data() -> ()  [unwired: 1 in, 2 out]
                  }
                  event "Ne": Value Change {
                    w2364 = u16 3 items=["ZERO", "AH", "DEC", "TUBO", "CUP"] ("Controlador")
                    n1825 = event-data() -> ()  [unwired: 1 in, 1 out]
                    n1826 = case shown="True" "Ne" {
                      tunnel: ["LAMP_NE" "LAMP_NE"] -> w2363
                      tunnel: ["DESLIGAR" "LIGAR"] -> w2362
                      frame False {
                      }
                      frame True {
                      }
                    }
                    n1827 = call "Monta Comando.vi"("Comando"=w2362, "Dispositivo"=w2363, "Controlador"=w2364) -> ()  [unwired: 4 in, 3 out]
                  }
                  event "He-Ar": Value Change {
                    w2372 = u16 3 items=["ZERO", "AH", "DEC", "TUBO", "CUP"] ("Controlador")
                    n1828 = event-data() -> ()  [unwired: 1 in, 1 out]
                    n1829 = case shown="False" "He-Ar" {
                      tunnel: ["LAMP_HE" "LAMP_HE"] -> w2371
                      tunnel: ["DESLIGAR" "LIGAR"] -> w2370
                      frame False {
                      }
                      frame True {
                      }
                    }
                    n1830 = call "Monta Comando.vi"("Comando"=w2370, "Dispositivo"=w2371, "Controlador"=w2372) -> ()  [unwired: 4 in, 3 out]
                  }
                  event "Sent_EspLampCass": Value Change {
                    w2380 = u16 3 items=["ZERO", "AH", "DEC", "TUBO", "CUP"] ("Controlador")
                    n1831 = event-data() -> ()  [unwired: 1 in, 1 out]
                    n1832 = property on="SlideEcass" class="Slide (strict)"("Visible"=TRUE) -> ()  [unwired: 2 in, 2 out]
                    n1833 = case shown="False" "Sent_EspLampCass" {
                      tunnel: ["ESP_LAMP" "ESP_LAMP"] -> w2379
                      tunnel: ["RECUAR" "AVANCAR"] -> w2378
                      frame False {
                      }
                      frame True {
                      }
                    }
                    n1834 = property on="stopEcass" class="Bool"("Visible"=FALSE) -> ()  [unwired: 2 in, 2 out]
                    n1835 = call "Monta Comando.vi"("Comando"=w2378, "Dispositivo"=w2379, "Controlador"=w2380) -> ()  [unwired: 4 in, 3 out]
                    "SlideEcass" <- u8 8 ("Slide")
                  }
                }
                n1836 = call "Bit Status TUBO.vi"("NomeStatus"=w2333) -> ("StatBit"=→"LedHe":bool)
                n1837 = call "Bit Status TUBO.vi"("NomeStatus"=w2334) -> ("StatBit"=→"LedNe":bool)
                n1838 = call "Bit Status TUBO.vi"("NomeStatus"=w2337) -> ("StatBit"=w2332:bool)
                n1839 = call "Bit Status TUBO.vi"("NomeStatus"=w2336) -> ("StatBit"=w2331:bool)
                n1840 = call "Bit Status TUBO.vi"("NomeStatus"=w2335) -> ("StatBit"=w2330:bool)
                n1841 = And(x=w2332, y=w2331) -> (x .and. y?=w2329:bool)
                "LedRep" <- w2329
                n1842 = And(x=w2332, y=w2330) -> (x .and. y?=w2328:bool)
                "LedCal" <- w2328
                n1843 = property on="SlideEcass" class="Slide (strict)"() -> ("Visible"=w2327:bool)  [unwired: 2 in, 2 out]
                n1844 = Or(x=w2329, y=w2328) -> (x .or. y?=w2339:bool)
                n1845 = Or(x=w2331, y=w2330) -> (x .or. y?=w2342:bool)
                n1846 = Not(x=w2332) -> (.not. x?=w2341:bool)
                n1847 = And(x=w2327, y=w2339) -> (x .and. y?=w2338:bool)
                n1848 = And(x=w2341, y=w2342) -> (x .and. y?=w2340:bool)
                n1849 = case shown="True" w2338 {
                  frame False {
                  }
                  frame True {
                    w2360 = u8 0 ("Disabled")
                    n1850 = property on="Sent_EspLampCass" class="Bool (strict)"("Disabled"=w2360) -> ()  [unwired: 2 in, 2 out]
                    n1851 = property on="He-Ar" class="Bool (strict)"("Disabled"=w2360) -> ()  [unwired: 2 in, 2 out]
                    n1852 = property on="Ne" class="Bool (strict)"("Disabled"=w2360) -> ()  [unwired: 2 in, 2 out]
                    n1853 = property on="SlideEcass" class="Slide (strict)"("Visible"=FALSE) -> ()  [unwired: 2 in, 2 out]
                  }
                }
                n1854 = case shown="True" w2340 {
                  frame False {
                  }
                  frame True {
                    w2344 = u8 2 ("Disabled")
                    n1855 = local read "SlideEcass"() -> (w2345:u8)
                    n1856 = property on="Sent_EspLampCass" class="Bool (strict)"("Disabled"=w2344) -> ()  [unwired: 2 in, 2 out]
                    n1857 = property on="Ne" class="Bool (strict)"("Disabled"=w2344) -> ()  [unwired: 2 in, 2 out]
                    n1858 = property on="He-Ar" class="Bool (strict)"("Disabled"=w2344) -> ()  [unwired: 2 in, 2 out]
                    n1859 = Add(x=w2345, y=u8 4) -> (x+y=w2347:u8)
                    n1860 = Greater Or Equal?(x=w2347, y=u8 100 ("x")) -> (x >= y?=w2348:bool)
                    n1861 = case shown="True" w2348 {
                      selector: w2348 -> [_ w2352]
                      tunnel: w2347 -> [w2351 _]
                      frame False {
                        n1862 = local write "SlideEcass"(w2351) -> ()
                        n1863 = property on="SlideEcass" class="Slide (strict)"("Fill Color"=u32 16750950 ("color(black)")) -> ()  [unwired: 2 in, 2 out]
                      }
                      frame True {
                        n1864 = local write "SlideEcass"(u8 92 ("Slide")) -> ()
                        n1865 = property on="stopEcass" class="Bool"("Visible"=w2352) -> ()  [unwired: 2 in, 2 out]
                        n1866 = property on="SlideEcass" class="Slide (strict)"("Fill Color"=u32 16724787 ("color(black)")) -> ()  [unwired: 2 in, 2 out]
                      }
                    }
                  }
                }
                n1867 = case shown="True" "stopEcass" {
                  frame False {
                  }
                  frame True {
                    w2359 = FALSE
                    w2358 = u8 0 ("Disabled")
                    w2357 = u16 3 items=["ZERO", "AH", "DEC", "TUBO", "CUP"] ("Controlador")
                    n1868 = call "Monta Comando.vi"("Comando"="DESLIGAR", "Dispositivo"="ESP_LAMP", "Controlador"=w2357) -> ()  [unwired: 4 in, 3 out]
                    n1869 = property on="Sent_EspLampCass" class="Bool (strict)"("Disabled"=w2358) -> ()  [unwired: 2 in, 2 out]
                    n1870 = property on="Ne" class="Bool (strict)"("Disabled"=w2358) -> ()  [unwired: 2 in, 2 out]
                    n1871 = property on="He-Ar" class="Bool (strict)"("Disabled"=w2358) -> ()  [unwired: 2 in, 2 out]
                    n1872 = property on="SlideEcass" class="Slide (strict)"("Visible"=w2359) -> ()  [unwired: 2 in, 2 out]
                    n1873 = property on="stopEcass" class="Bool"("Visible"=w2359) -> ()  [unwired: 2 in, 2 out]
                  }
                }
              }
              frame "Eucalyp." {
                # "Eucalyptus"
              }
              frame "Cam 1" {
                w2396 = 10
                w2403 = u16 15 items=["Alarme", "Atencao", "Erro", "Ocupado", "PosSecund", "PosConj#3", "MovFoco", "MovCjto#3", "Mov#4", "Mov#3", "Mov#2", "EspLamp", "HE", "NE", "EspLampRepouso", "EspLampCalibra"] ("NomeStatus")
                w2404 = u16 14 items=["Alarme", "Atencao", "Erro", "Ocupado", "PosSecund", "PosConj#3", "MovFoco", "MovCjto#3", "Mov#4", "Mov#3", "Mov#2", "EspLamp", "HE", "NE", "EspLampRepouso", "EspLampCalibra"] ("NomeStatus")
                w2405 = u16 11 items=["Alarme", "Atencao", "Erro", "Ocupado", "PosSecund", "PosConj#3", "MovFoco", "MovCjto#3", "Mov#4", "Mov#3", "Mov#2", "EspLamp", "HE", "NE", "EspLampRepouso", "EspLampCalibra"] ("NomeStatus")
                # "MUDANÇA:\nDESABILITA COMANDOS\nDE MOV. DO ESPELHO.\nRemover na implantação\ndefinitiva da CAM1."
                # "CAM 1"
                n1874 = event shown="[0] Timeout" {
                  selector: _ -> [_ _ _ _]
                  dyn-events: _ -> [_ _ _ _]
                  timeout: w2396 -> [_ _ _ _]
                  tunnel: ["timeout" ("Comando") w2422 w2428 w2434] -> w2389
                  event Timeout {
                    n1875 = event-data() -> ()  [unwired: 1 in, 2 out]
                  }
                  event "Mover/Parar": Value Change {
                    w2424 = u16 3 items=["ZERO", "AH", "DEC", "TUBO", "CUP"] ("Controlador")
                    n1876 = event-data() -> ("NewVal"=w2425:bool)  [unwired: 1 in, 4 out]
                    n1877 = case shown="True" w2425 {
                      tunnel: ["PARAR" ("Comando") "GIRAR" ("Comando")] -> w2422
                      frame False {
                      }
                      frame True {
                      }
                    }
                    n1878 = call "Monta Comando.vi"("Comando"=w2422, "Dispositivo"="ESP_CAMP", "Controlador"=w2424) -> ()  [unwired: 4 in, 3 out]
                  }
                  event "Sentido": Value Change {
                    w2429 = u16 3 items=["ZERO", "AH", "DEC", "TUBO", "CUP"] ("Controlador")
                    n1879 = event-data() -> ("NewVal"=w2431:bool)  [unwired: 1 in, 4 out]
                    n1880 = case shown="False" w2431 {
                      tunnel: ["RECUAR" "AVANCAR"] -> w2428
                      frame False {
                      }
                      frame True {
                      }
                    }
                    n1881 = call "Monta Comando.vi"("Comando"=w2428, "Dispositivo"="ESP_CAMP", "Controlador"=w2429) -> ()  [unwired: 4 in, 3 out]
                  }
                  event "Velocidade": Value Change {
                    w2436 = u16 3 items=["ZERO", "AH", "DEC", "TUBO", "CUP"] ("Controlador")
                    n1882 = event-data() -> ("NewVal"=w2437:bool)  [unwired: 1 in, 4 out]
                    n1883 = case shown="True" w2437 {
                      tunnel: ["AUMENTAR" "DIMINUIR"] -> w2434
                      frame False {
                      }
                      frame True {
                      }
                    }
                    n1884 = call "Monta Comando.vi"("Comando"=w2434, "Dispositivo"="ESP_CAMP", "Controlador"=w2436) -> ()  [unwired: 4 in, 3 out]
                  }
                }
                "Comando" <- w2389
                n1885 = case shown="False" "Sentido" {
